vi "ParGetStatus.vi"(0 "ref in":u64, 11 "error in (no error)":errorcluster) -> (4 "ref out":u64, 6 "Result":i32, 8 "Status":i32, 15 "error out":errorcluster)   [LabVIEW 2016, in "Snap7.lvlib"]
uses:
  Snap7.lvlib
  win32/lv_snap7.dll
panel:
  in  "var status":i32
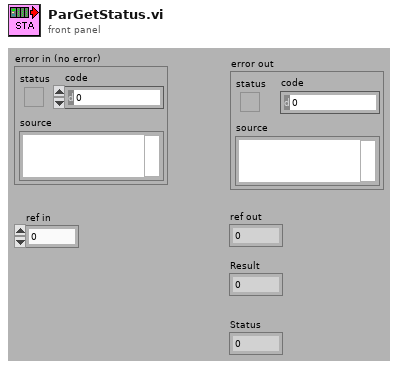
[diagram p1: front panel]
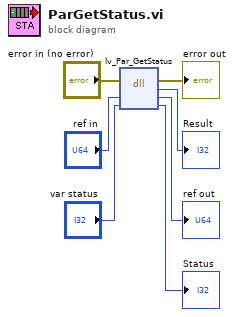
[diagram p0: block diagram]
diagram:
  n1 = dll-call lib="D:/maszup/svn/LineTraceSystem/SOFTWARE/sources/Drivers/PLC/Snap7/lib/win32/lv_snap7.dll" fn="lv_Par_GetStatus"(error in="error in (no error)", "Partner"="ref in", "Status"="var status") -> (error out=→"error out":errorcluster, "return type"=→"Result":i32, "Partner"=→"ref out":u64, "Status"=→"Status":i32)  [unwired: 2 in, 1 out]
